vi "Ticks per decisecond to Feet per second.vi"(11 "Drive Velocities (ticks/ds)":T1) -> (3 "Drive Velocities (ft/s)":T1)   [LabVIEW 2020]
doc: "converts ticks per decisecond (falcon units) to feet per second"
uses:
  Swerve Robot Project Template/Framework/Robot Global Data.vi
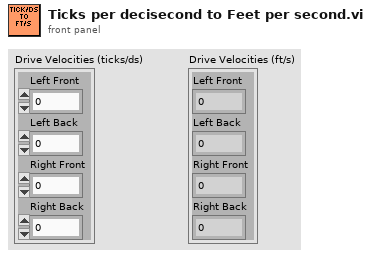
[diagram p1: front panel]
types:
  T1 = cluster{"Left Front":dbl, "Left Back":dbl, "Right Front":dbl, "Right Back":dbl}
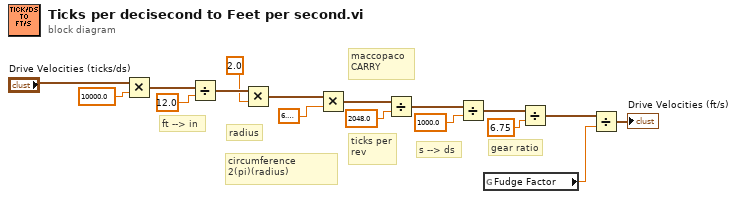
[diagram p0: block diagram]
diagram:
  # "s --> ds"
  # "circumference\n2(pi)(radius)"
  # "ticks per\nrev"
  # "ft --> in"
  # "radius"
  # "gear ratio"
  # "maccopaco\nCARRY"
  n1 = Multiply(x="Drive Velocities (ticks/ds)", y=10000.0) -> (x*y=w16:T1)
  n2 = Divide(x=w16, y=12.0) -> (x/y=w14:T1)
  n3 = Multiply(x=w14, y=2.0) -> (x*y=w12:T1)
  n4 = Multiply(x=w12, y=6.283185307179586) -> (x*y=w11:T1)
  n5 = Divide(x=w11, y=2048.0) -> (x/y=w9:T1)
  n6 = Divide(x=w9, y=1000.0) -> (x/y=w7:T1)
  n7 = global read "Robot Global Data.vi" "Fudge Factor"() -> (w2:dbl)
  n8 = Divide(x=w7, y=6.75) -> (x/y=w3:T1)
  n9 = Divide(x=w3, y=w2) -> (x/y=→"Drive Velocities (ft/s)":T1)
